vi "Last_samples (SubVI).vi"(9 "Array length":i32, 10 "Array in":sgl[](array[numeric]), 11 "Samples in":dbl[](array[numeric])) -> (3 "Array out":sgl[](array[numeric]))   [LabVIEW 2015]
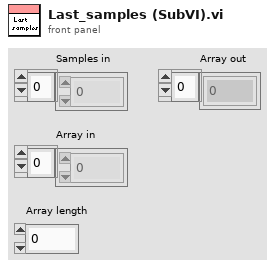
[diagram p1: front panel]
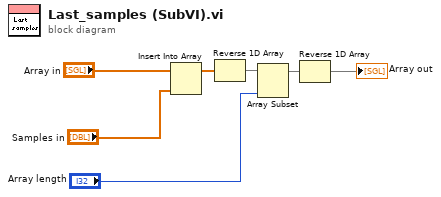
[diagram p0: block diagram]
diagram:
  n1 = Insert Into Array(array="Array in", new element="Samples in") -> (w4:sgl[])  [unwired: 1 in]
  n2 = Reverse 1D Array(array=w4) -> (reversed array=w6:sgl[])
  n3 = Array Subset(array=w6, length="Array length") -> (w7:sgl[])  [unwired: 1 in]
  n4 = Reverse 1D Array(array=w7) -> (reversed array=→"Array out":sgl[])
